vi "async initiate stop.vi"(8 "error in":errorcluster, 11 "module data in":T1={"run state"=enum."sync", "module"=refnum, "module ref"=refnum, "async exec ref"={"command fifo"=refnum, "error fifo"=refnum, "VI Refnum"=refnum, "input buffer"=refnum, "output buffer"=refnum, "process buffer"=refnum, "original dvrs"=[]}, "configuration ref"=refnum, "error"={"status"=FALSE, "code"=0, "source"=""}, "previous error code"=0, "input method"={"data table"={"Double"=[], "Single"=[], "I64"=[], "I32"=[], "I16"=[], "I8"=[], "U64"=[], "U32"=[], "U16"=[], "U8"=[], "Boolean"=[], "String"=[], "Array of Double"=[], "Array of Single"=[], "Array of I64"=[], "Array of I32"=[], "Array of I16"=[], "Array of I8"=[], "Array of U64"=[], "Array of U32"=[], "Array of U16"=[], "Array of U8"=[], "Array of Boolean"=[], "Array of String"=[]}, "transfer spec"=[]}, "output method"={"data table"={"Double"=[], "Single"=[], "I64"=[], "I32"=[], "I16"=[], "I8"=[], "U64"=[], "U32"=[], "U16"=[], "U8"=[], "Boolean"=[], "String"=[], "Array of Double"=[], "Array of Single"=[], "Array of I64"=[], "Array of I32"=[], "Array of I16"=[], "Array of I8"=[], "Array of U64"=[], "Array of U32"=[], "Array of U16"=[], "Array of U8"=[], "Array of Boolean"=[], "Array of String"=[]}, "transfer spec"=[]}, "process method parameters"={"data table"={"Double"=[], "Single"=[], "I64"=[], "I32"=[], "I16"=[], "I8"=[], "U64"=[], "U32"=[], "U16"=[], "U8"=[], "Boolean"=[], "String"=[], "Array of Double"=[], "Array of Single"=[], "Array of I64"=[], "Array of I32"=[], "Array of I16"=[], "Array of I8"=[], "Array of U64"=[], "Array of U32"=[], "Array of U16"=[], "Array of U8"=[], "Array of Boolean"=[], "Array of String"=[]}, "transfer spec"=[]}, "process method results"={"data table"={"Double"=[], "Single"=[], "I64"=[], "I32"=[], "I16"=[], "I8"=[], "U64"=[], "U32"=[], "U16"=[], "U8"=[], "Boolean"=[], "String"=[], "Array of Double"=[], "Array of Single"=[], "Array of I64"=[], "Array of I32"=[], "Array of I16"=[], "Array of I8"=[], "Array of U64"=[], "Array of U32"=[], "Array of U16"=[], "Array of U8"=[], "Array of Boolean"=[], "Array of String"=[]}, "transfer spec"=[]}, "fault handling"={"unknown"=[], "trivial"=[], "critical"=[], "recoverable"=[]}, "error report index "=-1}) -> (0 "error out":errorcluster, 3 "module data out":T1={"run state"=enum."sync", "module"=refnum, "module ref"=refnum, "async exec ref"={"command fifo"=refnum, "error fifo"=refnum, "VI Refnum"=refnum, "input buffer"=refnum, "output buffer"=refnum, "process buffer"=refnum, "original dvrs"=[]}, "configuration ref"=refnum, "error"={"status"=FALSE, "code"=0, "source"=""}, "previous error code"=0, "input method"={"data table"={"Double"=[], "Single"=[], "I64"=[], "I32"=[], "I16"=[], "I8"=[], "U64"=[], "U32"=[], "U16"=[], "U8"=[], "Boolean"=[], "String"=[], "Array of Double"=[], "Array of Single"=[], "Array of I64"=[], "Array of I32"=[], "Array of I16"=[], "Array of I8"=[], "Array of U64"=[], "Array of U32"=[], "Array of U16"=[], "Array of U8"=[], "Array of Boolean"=[], "Array of String"=[]}, "transfer spec"=[]}, "output method"={"data table"={"Double"=[], "Single"=[], "I64"=[], "I32"=[], "I16"=[], "I8"=[], "U64"=[], "U32"=[], "U16"=[], "U8"=[], "Boolean"=[], "String"=[], "Array of Double"=[], "Array of Single"=[], "Array of I64"=[], "Array of I32"=[], "Array of I16"=[], "Array of I8"=[], "Array of U64"=[], "Array of U32"=[], "Array of U16"=[], "Array of U8"=[], "Array of Boolean"=[], "Array of String"=[]}, "transfer spec"=[]}, "process method parameters"={"data table"={"Double"=[], "Single"=[], "I64"=[], "I32"=[], "I16"=[], "I8"=[], "U64"=[], "U32"=[], "U16"=[], "U8"=[], "Boolean"=[], "String"=[], "Array of Double"=[], "Array of Single"=[], "Array of I64"=[], "Array of I32"=[], "Array of I16"=[], "Array of I8"=[], "Array of U64"=[], "Array of U32"=[], "Array of U16"=[], "Array of U8"=[], "Array of Boolean"=[], "Array of String"=[]}, "transfer spec"=[]}, "process method results"={"data table"={"Double"=[], "Single"=[], "I64"=[], "I32"=[], "I16"=[], "I8"=[], "U64"=[], "U32"=[], "U16"=[], "U8"=[], "Boolean"=[], "String"=[], "Array of Double"=[], "Array of Single"=[], "Array of I64"=[], "Array of I32"=[], "Array of I16"=[], "Array of I8"=[], "Array of U64"=[], "Array of U32"=[], "Array of U16"=[], "Array of U8"=[], "Array of Boolean"=[], "Array of String"=[]}, "transfer spec"=[]}, "fault handling"={"unknown"=[], "trivial"=[], "critical"=[], "recoverable"=[]}, "error report index "=-1})   [LabVIEW 2013, in "main engine.lvlib"]
uses:
  main engine/main engine.lvlib
  main engine/full module data.ctl
  <vilib>/NI/Tag Bus Module Framework/runtime/TBM module execution interface.lvclass
  main engine/module run state.ctl
  asynchronous executor reference.ctl
  async message to executor.ctl
  Runtime/async command notification.ctl
  <vilib>/NI/Tag Bus/table/data table.ctl
  Runtime/async error info.ctl
  <vilib>/NI/Tag Bus Module Framework/runtime/error classification.ctl
  <vilib>/NI/Tag Bus Module Framework/module configuration/TBM module configuration.lvclass
  main engine/module method data.ctl
  <vilib>/NI/Tag Bus/table/transfer specification.ctl
  <vilib>/NI/Tag Bus/tag/Data Type.ctl
  main engine/fault handling spec.ctl
  Configuration/Error Actions.ctl
  <vilib>/NI/Tag Bus/table/data table.lvlib
  <vilib>/NI/Tag Bus/tag/tag descriptor.lvclass
  Configuration/Standard Engine Configuration.lvclass
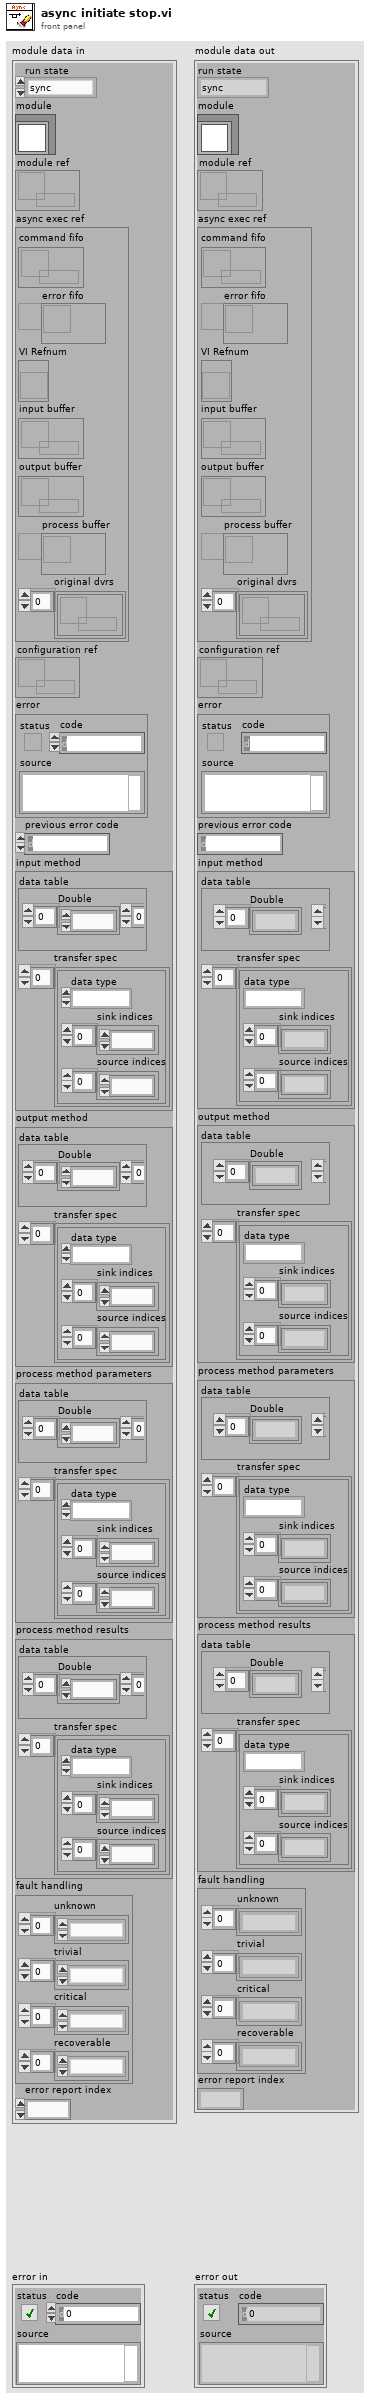
[diagram p1: front panel]
types:
  T1 = typedef "main engine.lvlib/full module data.ctl" = cluster{"run state":T2, "module":refnum<class "TBM module execution interface.lvclass">, "module ref":refnum<data-value>, "async exec ref":T3, "configuration ref":refnum<data-value>, "error":errorcluster, "previous error code":i32, "input method":T4, "output method":T4, "process method parameters":T4, "process method results":T4, "fault handling":T8, "error report index ":i32}
  T2 = typedef "main engine.lvlib/module run state.ctl" = enum16{"sync", "async"}
  T3 = typedef "main engine.lvlib/asynchronous executor reference.ctl" = cluster{"command fifo":refnum<k33>, "error fifo":refnum<k33>, "VI Refnum":refnum<vi>, "input buffer":refnum<k33>, "output buffer":refnum<k33>, "process buffer":refnum<k33>, "original dvrs":refnum<data-value>[]}
  T4 = typedef "main engine.lvlib/module method data.ctl" = cluster{"data table":T5, "transfer spec":T6[]}
  T5 = typedef "tag bus.lvlib/data table.lvlib/data table.ctl" = cluster{"Double":dbl[], "Single":sgl[], "I64":i64[], "I32":i32[], "I16":i16[], "I8":i8[], "U64":u64[], "U32":u32[], "U16":u16[], "U8":u8[], "Boolean":bool[], "String":string[], "Array of Double":cluster{"DBL Array":dbl[]}[], "Array of Single":cluster{"SGL Array":sgl[]}[], "Array of I64":cluster{"I64 Array":i64[]}[], "Array of I32":cluster{"I32 Array":i32[]}[], "Array of I16":cluster{"I16 Array":i16[]}[], "Array of I8":cluster{"I8 Array":i8[]}[], "Array of U64":cluster{"U64 Array":u64[]}[], "Array of U32":cluster{"U32 Array":u32[]}[], "Array of U16":cluster{"U16 Array":u16[]}[], "Array of U8":cluster{"U8 Array":u8[]}[], "Array of Boolean":cluster{"Boolean Array":bool[]}[], "Array of String":cluster{"String Array":string[]}[]}
  T6 = typedef "tag bus.lvlib/data table.lvlib/transfer specification.ctl" = cluster{"data type":T7, "sink indices":i32[], "source indices":i32[]}
  T7 = typedef "tag bus.lvlib/tag descriptor.lvclass/Data Type.ctl" = enum16{"Double", "Single", "I64", "I32", "I16", "I8", "U64", "U32", "U16", "U8", "Boolean", "String", "Array of Double", "Array of Single", "Array of I64", "Array of I32", "Array of I16", "Array of I8", "Array of U64", "Array of U32", "Array of U16", "Array of U8", "Array of Boolean", "Array of String"}
  T8 = typedef "main engine.lvlib/fault handling spec.ctl" = cluster{"unknown":T9[], "trivial":T9[], "critical":T9[], "recoverable":T9[]}
  T9 = typedef "Standard Engine Configuration.lvclass/Error Actions.ctl" = enum16{"Clear", "Notify", "Stop Component", "Stop Engine", "Safe State", "Attempt Recovery"}
  T10 = typedef "main engine.lvlib/async command notification.ctl" = enum16{"stop", "input", "process", "output"}
  T11 = typedef "main engine.lvlib/async message to executor.ctl" = cluster{"command":T10, "data 1 (i,o,pp)":refnum<data-value>, "data 2 (pr)":refnum<data-value>, "user value":u64}
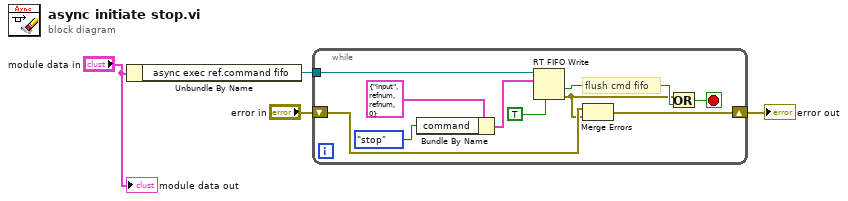
[diagram p0: block diagram]
diagram:
  n1 = Unbundle By Name("module data in") -> ("async exec ref.command fifo"=w3:refnum<k33>)
  n2 = while {
    tunnel: w3 -> [w14]
    shift-right: [w12] -> w1
    shift-left: "error in" -> [w11]
    stop <- w9 stop-if-true
    # "flush cmd fifo"
    n3 = Bundle By Name(cluster=T11 {"command"=enum."input", "data 1 (i,o,pp)"=refnum, "data 2 (pr)"=refnum, "user value"=0} ("element"), "command"=async_command_notification."stop") -> (w6:T11)
    n4 = RT FIFO Write(0:w14, 1:w6, 5:TRUE ("overwrite on timeout (T)")) -> (10:w10:bool, 11:w8:errorcluster)  [unwired: 2 in, 2 out]
    n5 = Merge Errors(w11, w8) -> (w12:errorcluster)
    n6 = Or(x=w8, y=w10) -> (x .or. y?=w9:bool)
  }
  "error out" <- w1
  "module data out" <- "module data in"
